vi "Find All Hardware Custom Devices.vi"(8 "error in (no error)":errorcluster, 11 "Routing and Faulting Ref in":T1 format="%.0x") -> (0 "error out":errorcluster, 2 "Hardware Refs":T1[](array[typedef]) format="%.0x", 3 "Routing and Faulting Ref out":T1 format="%.0x")   [LabVIEW 2020, in "Routing and Faulting Hardware API.lvlib"]
uses:
  Routing and Faulting Hardware API.lvlib
  <vilib>/NI VeriStand/Custom Device API/Custom Device Item Ref.ctl
  Routing and Faulting Hardware API Constants.vi
  <vilib>/NI VeriStand/Custom Device API/Custom Device API.lvlib
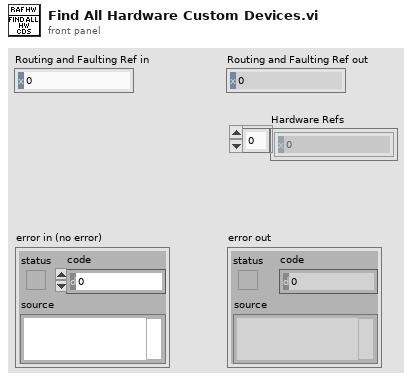
[diagram p1: front panel]
types:
  T1 = typedef "Custom Device API.lvlib/Custom Device Item Ref.ctl" = u64
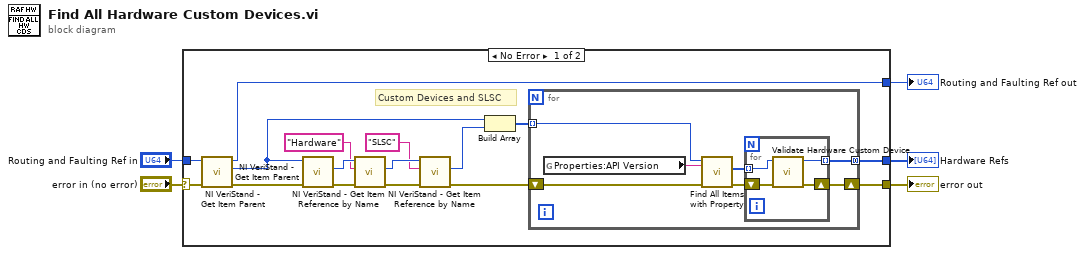
[diagram p0: block diagram]
diagram:
  n1 = case shown="No Error" "error in (no error)" {
    selector: "error in (no error)" -> [w16 w34]
    tunnel: [w21 w34] -> w4
    tunnel: "Routing and Faulting Ref in" -> [w15 w33]
    tunnel: [w14 w33] -> w2
    tunnel: [w20 _] -> w1
    frame No Error {
      # "Custom Devices and SLSC"
      n2 = call <vilib>:"NI VeriStand - Get Item Parent.vi"("error in (no error)"=w16, "Item Ref in"=w15) -> ("error out"=w19:errorcluster, "Parent Ref"=w8:T1, "Item Ref out"=w14:T1)  [unwired: 6 in, 1 out]
      n3 = call <vilib>:"NI VeriStand - Get Item Parent.vi"("error in (no error)"=w19, "Item Ref in"=w8) -> ("error out"=w17:errorcluster, "Parent Ref"=w18:T1)  [unwired: 6 in, 2 out]
      n4 = call <vilib>:"NI VeriStand - Get Item Reference by Name.vi"("error in (no error)"=w17, "Item Name"="Hardware", "Parent Ref in"=w18) -> ("error out"=w7:errorcluster, "Item Ref"=w12:T1)  [unwired: 5 in, 2 out]
      n5 = call <vilib>:"NI VeriStand - Get Item Reference by Name.vi"("error in (no error)"=w7, "Item Name"="SLSC", "Parent Ref in"=w12) -> ("error out"=w6:errorcluster, "Item Ref"=w11:T1)  [unwired: 5 in, 2 out]
      n6 = Build Array(w8, w11) -> (w13:T1[])
      n7 = for {
        tunnel: [w27] -> w20 mode=concatenating
        tunnel: w13 -> [w25] mode=indexing
        shift-right: [w28] -> w21
        shift-left: w6 -> [w26]
        n8 = global read "Routing and Faulting Hardware API Constants.vi" "Properties:API Version"() -> (w22:string)
        n9 = call "Find All Items with Property.vi"("error in"=w26, "Property Name"=w22, "Section Ref in"=w25) -> ("error out"=w24:errorcluster, "Item Refs"=w23:T1[])  [unwired: 5 in, 2 out]
        n10 = for {
          shift-right: [w30] -> w28
          shift-left: w24 -> [w29]
          tunnel: [w32] -> w27 mode=indexing
          tunnel: w23 -> [w31] mode=indexing
          n11 = call "Validate Hardware Custom Device.vi"("error in (no error)"=w29, "Hardware Ref in"=w31) -> ("error out"=w30:errorcluster, "Hardware Ref out"=w32:T1)  [unwired: 8 in]
        }
      }
    }
    frame Error {
    }
  }
  "Routing and Faulting Ref out" <- w2
  "error out" <- w4
  "Hardware Refs" <- w1
